vi "Measure all pixels on cell and save data.vi"(0 "Cell details cluster in":T1={"Measure?"=TRUE, "Area (cm^2)"=0.0, "Cell Label"="", "Cell Description"="", "Cell Position"=0, "Time in rig (s)"=0.0, "Time to next scan (s)"=0.0, "Scan number"=0.0, "When did you stick it in?"=0.0, "Time between scans (s)"=0.0, "Time of the last scan (s)"=0.0, "Scan settings in queue"=0, "Sample Holder"=0.0} {"Scan settings in queue" items=["Regular", "Inverted"]; "Time of the last scan (s)" format="%<%H:%M:%S>t"; "When did you stick it in?" format="%<%H:%M:%S>t"; "Time to next scan (s)" format="%<%H:%M:%S>t"; "Time in rig (s)" format="%<%H:%M:%S>t"}, 1 "Username":string, 5 "Cell Description":string, 6 "XYGraph Refnum":refnum<vi>, 7 "Cell position":dbl, 8 "Tbl Refnum":refnum<vi>, 9 "Sample Holder":dbl, 11 "Scan settings in queue":dbl, 12 "JV curve scan settings":T2(array[cluster])=[{"Light Intensity (Suns)"=1.0, "Stabilization Time (s)"=2.0, "Maximum Voltage (V)"=0.0, "Minimum Voltage (V)"=-1.4, "Range Options"=0, "Scan Direction\nDU (T), UD (F)"=FALSE, "Step Size (V)"=0.01, "Source Delay (s)"=0.001}, {"Light Intensity (Suns)"=1.0, "Stabilization Time (s)"=5.0, "Maximum Voltage (V)"=2.0, "Minimum Voltage (V)"=0.0, "Range Options"=0, "Scan Direction\nDU (T), UD (F)"=TRUE, "Step Size (V)"=0.04, "Source Delay (s)"=0.001}] {"Range Options" items=["Auto Range", "Semi-Auto Range", "100 uA", "1 mA", "10 mA", "100 mA", "1A"]}, 13 "Time Zero":timestamp) -> (4 "Cell details cluster out":T1={"Measure?"=TRUE, "Area (cm^2)"=0.0, "Cell Label"="", "Cell Description"="", "Cell Position"=0, "Time in rig (s)"=0.0, "Time to next scan (s)"=0.0, "Scan number"=0.0, "When did you stick it in?"=0.0, "Time between scans (s)"=0.0, "Time of the last scan (s)"=0.0, "Scan settings in queue"=0, "Sample Holder"=0.0} {"Scan settings in queue" items=["Regular", "Inverted"]; "Time of the last scan (s)" format="%<%H:%M:%S>t"; "When did you stick it in?" format="%<%H:%M:%S>t"; "Time to next scan (s)" format="%<%H:%M:%S>t"; "Time in rig (s)" format="%<%H:%M:%S>t"}, 15 "JV curve image path":path)   [LabVIEW 2011]
uses:
  <vilib>/ULx/Create Channel.llb/ULx Create Channel (DO-Digital Output).vi
  <vilib>/ULx/Write.llb/ULx Write (Digital U32 1Chan 1Samp).vi
  <instrlib>/Keithley 24XX/Keithley 24XX.lvlib
panel:
  in  "Tab Control 4":enum32{"Page 1"}(tab)
  out "JV Curve":cluster{"Y":dbl[], "Y":dbl[]}[](graph)
  in  "VISA resource name":refnum<visa-resource-name>="GPIB0::24::INSTR"
  in  "Port":refnum<k21>="Dev0/AuxPort"
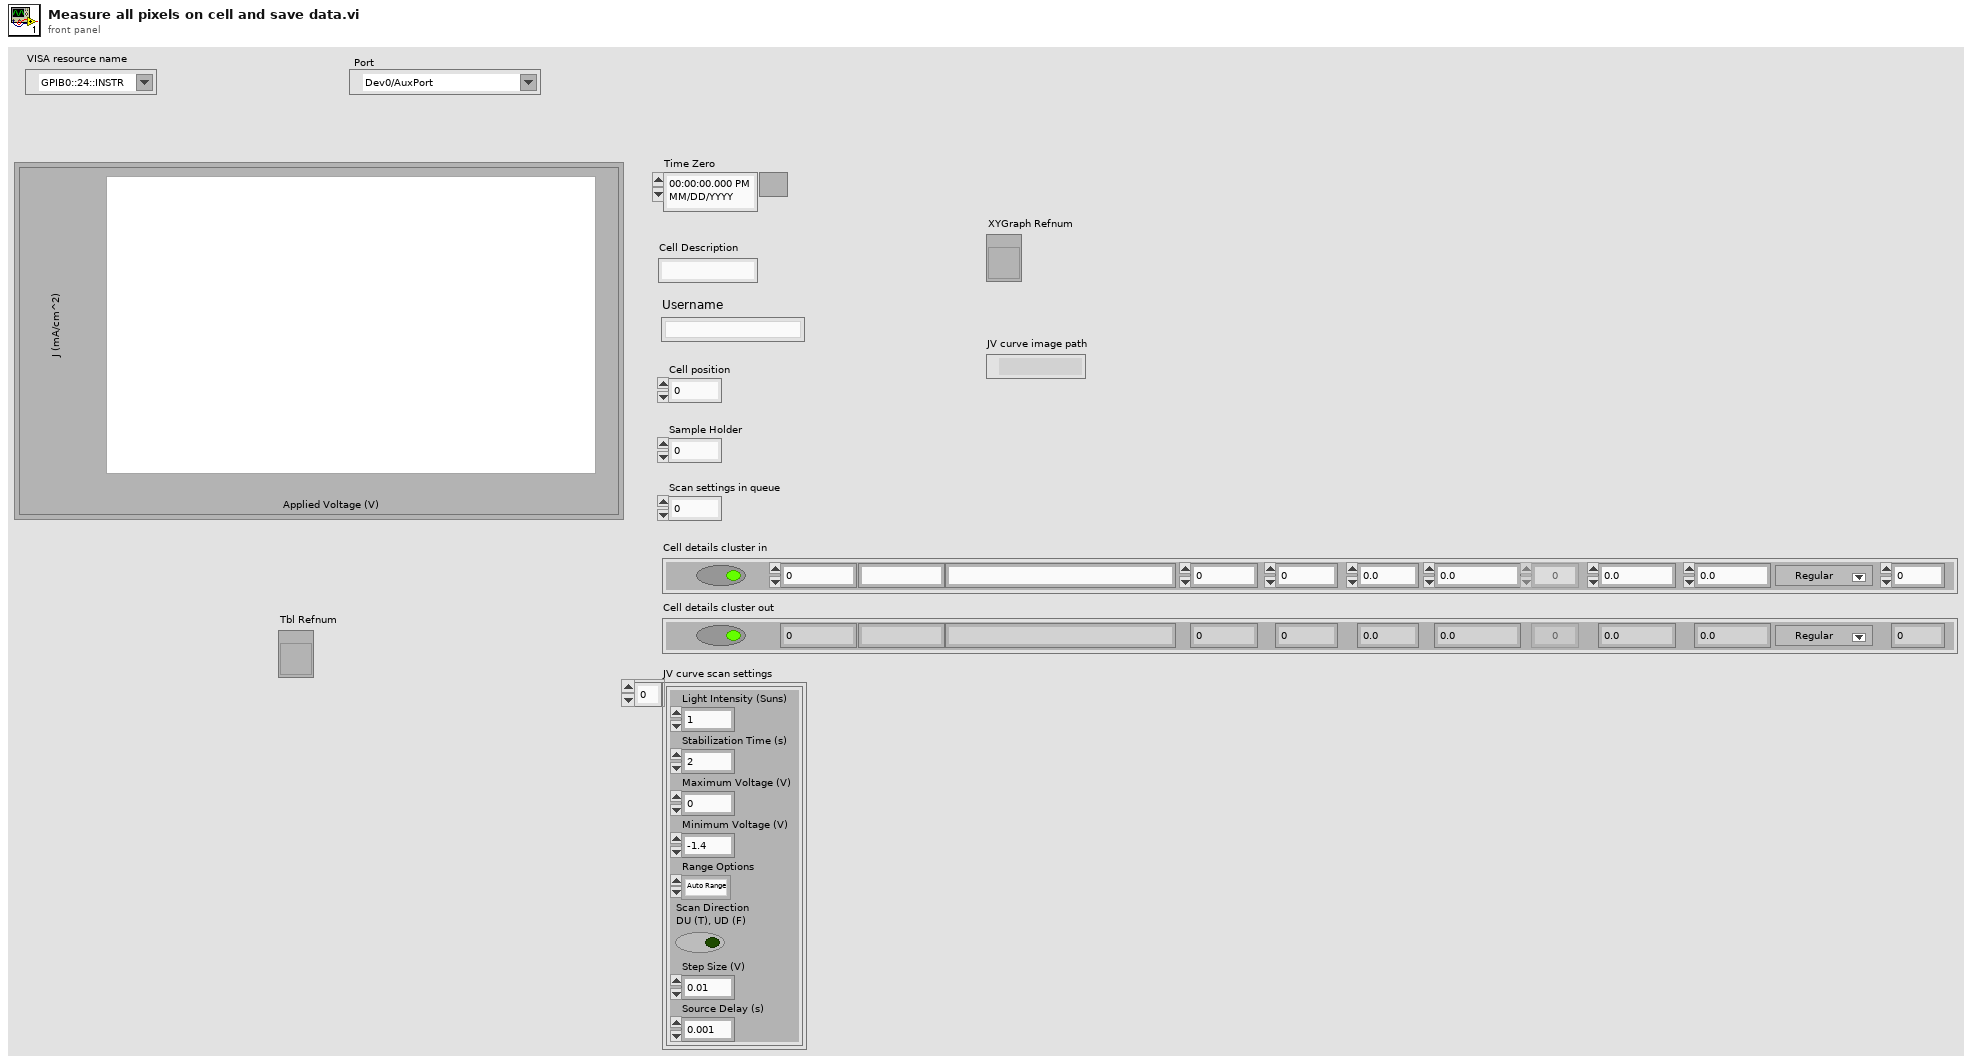
[diagram p1: front panel]
types:
  T1 = cluster{"Measure?":bool, "Area (cm^2)":dbl, "Cell Label":string, "Cell Description":string, "Cell Position":i32, "Time in rig (s)":dbl, "Time to next scan (s)":dbl, "Scan number":dbl, "When did you stick it in?":dbl, "Time between scans (s)":dbl, "Time of the last scan (s)":dbl, "Scan settings in queue":u16, "Sample Holder":dbl}
  T2 = cluster{"Light Intensity (Suns)":dbl, "Stabilization Time (s)":dbl, "Maximum Voltage (V)":dbl, "Minimum Voltage (V)":dbl, "Range Options":u16, "Scan Direction\nDU (T), UD (F)":bool, "Step Size (V)":dbl, "Source Delay (s)":dbl}[]
  T3 = cluster{"Light Intensity (Suns)":dbl, "Stabilization Time (s)":dbl, "Maximum Voltage (V)":dbl, "Minimum Voltage (V)":dbl, "Range Options":u16, "Scan Direction\nDU (T), UD (F)":bool, "Step Size (V)":dbl, "Source Delay (s)":dbl}
  T4 = typedef "imagedata.ctl" = cluster{"image type":i32, "image depth":i32, "image":u8[], "mask":u8[], "colors":u32[], "Rectangle":cluster{"left":i16, "top":i16, "right":i16, "bottom":i16}}
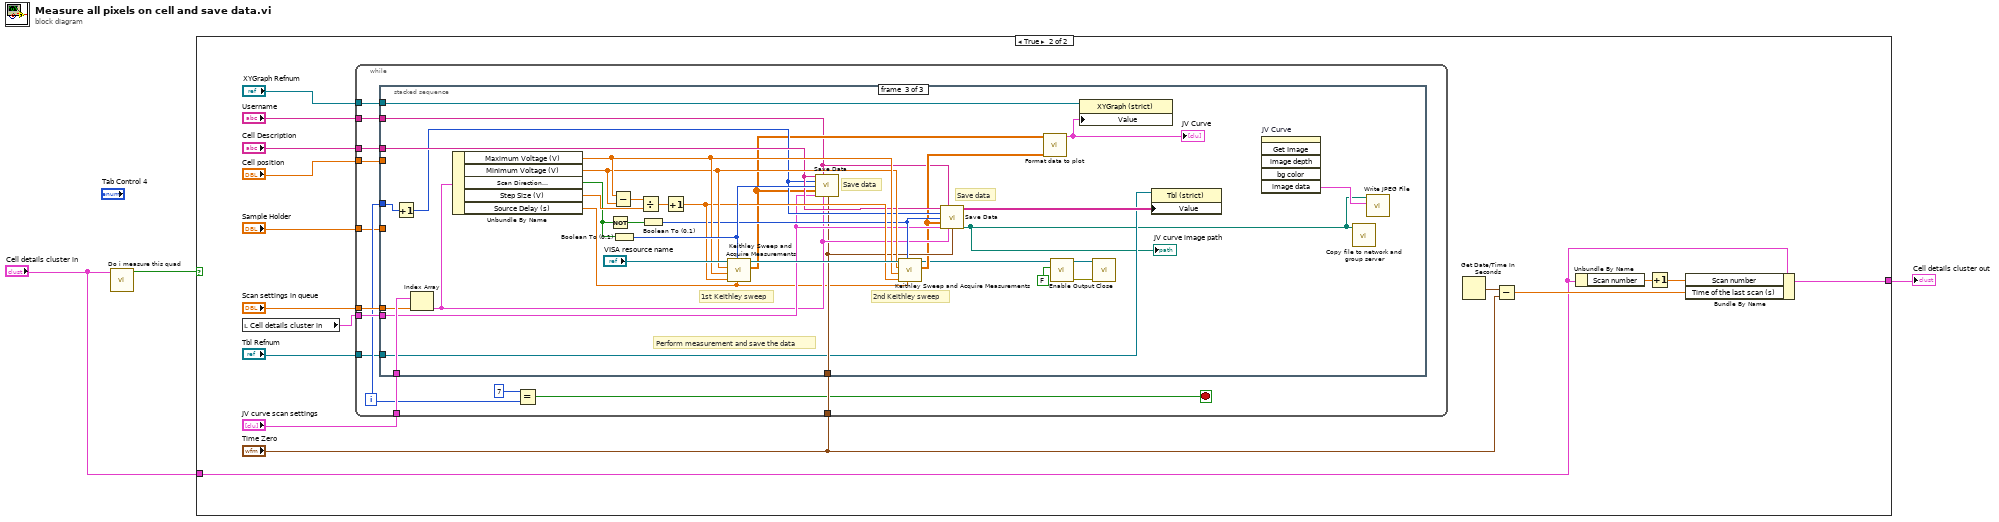
[diagram p0: block diagram]
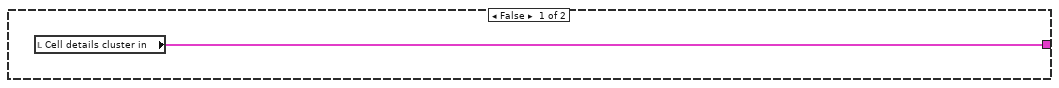
[diagram p2: hidden frame]
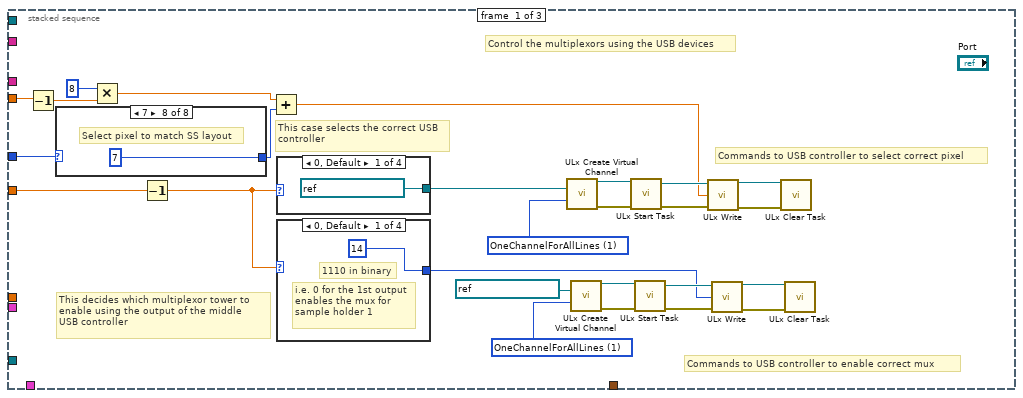
[diagram p3: hidden frame]
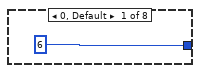
[diagram p4: hidden frame]
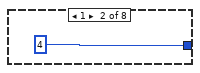
[diagram p5: hidden frame]
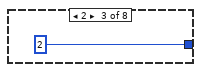
[diagram p6: hidden frame]
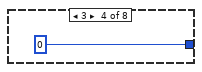
[diagram p7: hidden frame]
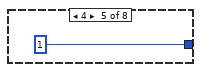
[diagram p8: hidden frame]
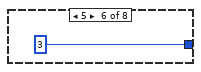
[diagram p9: hidden frame]
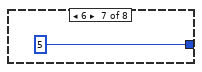
[diagram p10: hidden frame]
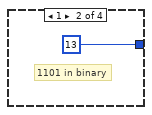
[diagram p11: hidden frame]
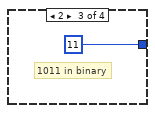
[diagram p12: hidden frame]
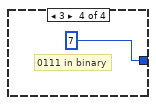
[diagram p13: hidden frame]
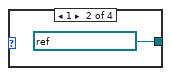
[diagram p14: hidden frame]
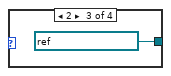
[diagram p15: hidden frame]
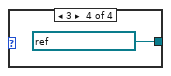
[diagram p16: hidden frame]
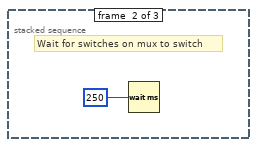
[diagram p17: hidden frame]
diagram:
  n1 = call "Do i measure this quad.vi"("Cell details"="Cell details cluster in") -> ("Measure cell?"=w3:bool)  [unwired: 10 in]
  n2 = case shown="True" w3 {
    tunnel: [w4 w9] -> w2
    tunnel: "Cell details cluster in" -> [_ w5]
    frame False {
      n3 = local read "Cell details cluster in"() -> (w4:T1)
    }
    frame True {
      n4 = local read "Cell details cluster in"() -> (w14:T1)
      n5 = while {
        tunnel: "JV curve scan settings" -> [w33]
        tunnel: "Scan settings in queue" -> [w32]
        tunnel: w14 -> [w31]
        tunnel: "Cell position" -> [w30]
        tunnel: "Sample Holder" -> [w27]
        tunnel: "Cell Description" -> [w26]
        tunnel: "Time Zero" -> [w25]
        tunnel: "Username" -> [w23]
        tunnel: "XYGraph Refnum" -> [w22]
        tunnel: "Tbl Refnum" -> [w21]
        i -> [w28]
        stop <- w24 stop-if-true
        n6 = stacked-sequence {
          tunnel: w33 -> [_ _ w109]
          tunnel: w32 -> [_ _ w108]
          tunnel: w31 -> [_ _ w93]
          tunnel: w30 -> [w49 _ _]
          tunnel: w28 -> [w35 _ w101]
          tunnel: w27 -> [w46 _ _]
          tunnel: w26 -> [_ _ w96]
          tunnel: w25 -> [_ _ w91]
          tunnel: w23 -> [_ _ w83]
          tunnel: w22 -> [_ _ w82]
          tunnel: w21 -> [_ _ w80]
          frame #0 {
            w45 = 1 items=["OneChannelForEachLine", "OneChannelForAllLines"] ("line grouping")
            w58 = 1 items=["OneChannelForEachLine", "OneChannelForAllLines"] ("line grouping")
            # "Control the multiplexors using the USB devices"
            # "Commands to USB controller to enable correct mux"
            # "Commands to USB controller to select correct pixel"
            # "This decides which multiplexor tower to\nenable using the output of the middle \nUSB controller"
            # "This case selects the correct USB\ncontroller"
            n7 = Decrement(x=w49) -> (x-1=w48:dbl)
            n8 = case shown="7" w35 {
              tunnel: [6 4 2 0 1 3 5 7] -> w34
              frame 0, Default {
              }
              frame 1 {
              }
              frame 2 {
              }
              frame 3 {
              }
              frame 4 {
              }
              frame 5 {
              }
              frame 6 {
              }
              frame 7 {
                # "Select pixel to match SS layout"
              }
            }
            n9 = Multiply(x=8, y=w48) -> (x*y=w50:dbl)
            n10 = Decrement(x=w46) -> (x-1=w37:dbl)
            n11 = Add(x=w50, y=w34) -> (x+y=w47:dbl)
            n12 = case shown="0, Default" w37 {
              tunnel: [refnum<k21> "Dev0/1stPortA" ("Port 2") refnum<k21> "Dev0/1stPortB" ("Port 2") refnum<k21> "Dev1/1stPortA" ("Port 2") refnum<k21> "Dev1/1stPortB" ("Port 2")] -> w59
              frame 0, Default {
              }
              frame 1 {
              }
              frame 2 {
              }
              frame 3 {
              }
            }
            n13 = case shown="0, Default" w37 {
              tunnel: [14 13 11 7] -> w36
              frame 0, Default {
                # "i.e. 0 for the 1st output\nenables the mux for\nsample holder 1"
                # "1110 in binary"
              }
              frame 1 {
                # "1101 in binary"
              }
              frame 2 {
                # "1011 in binary"
              }
              frame 3 {
                # "0111 in binary"
              }
            }
            n14 = call-poly <vilib>:"ULx Create Virtual Channel.vi"("lines"=w59, "line grouping"=w58) -> ("task out"=w56:refnum<k24>, "error out"=w57:errorcluster)  [unwired: 12 in]
            n15 = call-poly <vilib>:"ULx Create Virtual Channel.vi"("lines"=refnum<k21> "Dev2/1stPortA" ("Port 2"), "line grouping"=w45) -> ("task out"=w43:refnum<k24>, "error out"=w44:errorcluster)  [unwired: 12 in]
            n16 = call <vilib>:"ULx Start Task.vi"("task in"=w56, "error in"=w57) -> ("task out"=w53:refnum<k24>, "error out"=w52:errorcluster)  [unwired: 12 in]
            n17 = call <vilib>:"ULx Start Task.vi"("task in"=w43, "error in"=w44) -> ("task out"=w40:refnum<k24>, "error out"=w39:errorcluster)  [unwired: 12 in]
            n18 = call-poly <vilib>:"ULx Write.vi"("task in"=w53, "data"=w47, "error in"=w52) -> ("task out"=w55:refnum<k24>, "error out"=w54:errorcluster)  [unwired: 10 in, 1 out]
            n19 = call-poly <vilib>:"ULx Write.vi"("task in"=w40, "data"=w36, "error in"=w39) -> ("task out"=w42:refnum<k24>, "error out"=w41:errorcluster)  [unwired: 10 in, 1 out]
            n20 = call <vilib>:"ULx Clear Task.vi"("task in"=w55, "error in"=w54) -> ()  [unwired: 13 in, 1 out]
            n21 = call <vilib>:"ULx Clear Task.vi"("task in"=w42, "error in"=w41) -> ()  [unwired: 13 in, 1 out]
          }
          frame #1 {
            # "Wait for switches on mux to switch"
            n22 = Wait (ms)(milliseconds to wait=250) -> ()  [unwired: 1 out]
          }
          frame #2 {
            # "Perform measurement and save the data"
            # "Save data"
            # "Save data"
            # "2nd Keithley sweep"
            # "1st Keithley sweep"
            n23 = Increment(x=w101) -> (x+1=w95:i32)
            n24 = Index Array(array=w109, index=w108) -> (element=w92:T3)
            n25 = Unbundle By Name(w92) -> ("Maximum Voltage (V)"=w99:dbl, "Minimum Voltage (V)"=w98:dbl, "Scan Direction\nDU (T), UD (F)"=w103:bool, "Step Size (V)"=w105:dbl, "Source Delay (s)"=w90:dbl)
            n26 = Not(x=w103) -> (.not. x?=w104:bool)
            n27 = Subtract(x=w99, y=w98) -> (x-y=w106:dbl)
            n28 = Boolean To (0,1)(Boolean=w103) -> (0, 1=w102:i16)
            n29 = Divide(x=w106, y=w105) -> (x/y=w107:dbl)
            n30 = Boolean To (0,1)(Boolean=w104) -> (0, 1=w94:i16)
            n31 = Increment(x=w107) -> (x+1=w97:dbl)
            n32 = call "Keithley Sweep and Acquire Measurements.vi"("Source Delay (s)"=w90, "Sweep Direction"=w102, "Number of Points"=w97, "Maximum Amplitude"=w99, "Minimum Amplitude"=w98, "VISA resource name"="VISA resource name") -> ("Data Array"=w89:dbl[][], "VISA resource name out"=w100:refnum<visa-resource-name>)  [unwired: 1 in, 1 out]
            n33 = call "Save Data.vi"("Experiment Indicator"=w96, "Username"=w83, "Pixel"=w95, "Scan direction"=w102, "Data Array"=w89, "Cell details cluster"=w93, "Show me Scan \nSettings JV set"=w92, "Time zero"=w91) -> ()  [unwired: 3 in, 5 out]
            n34 = call "Keithley Sweep and Acquire Measurements.vi"("Source Delay (s)"=w90, "Sweep Direction"=w94, "Number of Points"=w97, "Maximum Amplitude"=w99, "Minimum Amplitude"=w98, "VISA resource name"=w100) -> ("Data Array"=w88:dbl[][], "VISA resource name out"=w87:refnum<visa-resource-name>)  [unwired: 1 in, 1 out]
            n35 = call "Save Data.vi"("Experiment Indicator"=w96, "Username"=w83, "Pixel"=w95, "Scan direction"=w94, "Data Array"=w88, "Cell details cluster"=w93, "Show me Scan \nSettings JV set"=w92, "Time zero"=w91) -> ("Master Log"=w81:string[][], "File path for JV image"=w77:path)  [unwired: 3 in, 3 out]
            "JV curve image path" <- w77
            n36 = call "Format data to plot.vi"("Data Array 2"=w88, "Data Array"=w89) -> ("JV Curve"=w79:cluster{"Y":dbl[], "Y":dbl[]}[])  [unwired: 9 in]
            "JV Curve" <- w79
            n37 = call <instrlib>:"Enable Output.vi"("Enable Output (T: Enable)"=FALSE, "VISA resource name"=w87) -> ("error out"=w85:errorcluster, "VISA resource name out"=w86:refnum<visa-resource-name>)  [unwired: 8 in]
            n38 = property class="XYGraph (strict)"(reference=w82, "Value"=w79) -> ()  [unwired: 1 in, 2 out]
            n39 = call <instrlib>:"Close.vi"("error in (no error)"=w85, "VISA resource name"=w86) -> ()  [unwired: 9 in, 1 out]
            n40 = property class="Tbl (strict)"(reference=w80, "Value"=w81) -> ()  [unwired: 1 in, 2 out]
            n41 = invoke on="JV Curve" class="XYGraph (strict)" method="Get Image"() -> ("image data"=w78:T4)  [unwired: 6 in, 5 out]
            n42 = call "Copy file to network and group server.vi"("File path in"=w77) -> ()  [unwired: 11 in]
            n43 = call <vilib>:"Write JPEG File.vi"("image data"=w78, "path to JPEG file"=w77) -> ()  [unwired: 8 in, 2 out]
          }
        }
        n44 = Equal?(x=7, y=w28) -> (x = y?=w24:bool)
      }
      n45 = Get Date/Time In Seconds() -> (seconds since 1Jan1904=w13:timestamp)
      n46 = Subtract(x=w13, y="Time Zero") -> (x-y=w8:dbl)
      n47 = Unbundle By Name(w5) -> ("Scan number"=w10:dbl)
      n48 = Increment(x=w10) -> (x+1=w11:dbl)
      n49 = Bundle By Name(cluster=w5, "Scan number"=w11, "Time of the last scan (s)"=w8) -> (w9:T1)
    }
  }
  "Cell details cluster out" <- w2
